vi "SerialPort.Get Status.vi"(8 "error in (no error)":errorcluster, 11 "SerialPort in":refnum<class "SerialPort.lvclass">) -> (0 "error out":errorcluster, 2 "State":T1, 3 "SerialPort out":refnum<class "SerialPort.lvclass">)   [LabVIEW 2018, in "SerialPort.lvclass"]
uses:
  SerialPort.lvclass
  Controls/SerialPort.Status Enum.ctl
  SerialPort.lvclass/SerialPort.ctl
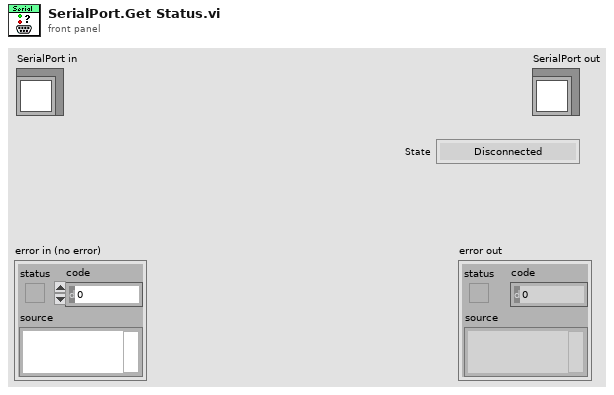
[diagram p1: front panel]
types:
  T1 = typedef "SerialPort.Status Enum.ctl" = enum16{"Disconnected", "Connecting", "Connected"}
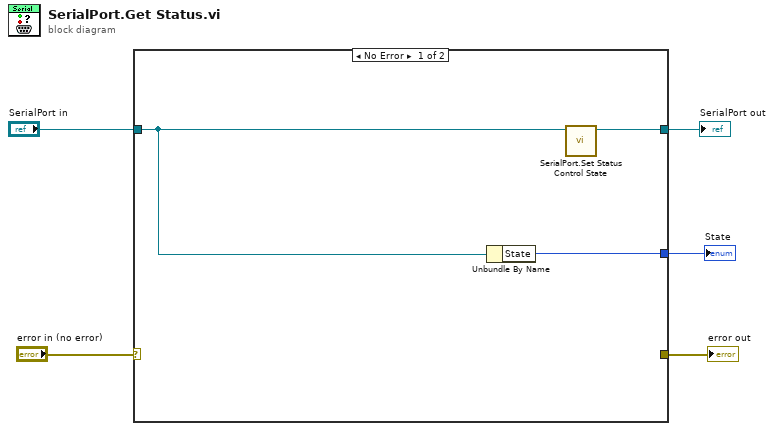
[diagram p0: block diagram]
diagram:
  n1 = case shown="No Error" "error in (no error)" {
    selector: "error in (no error)" -> [_ w10]
    tunnel: [_ w10] -> w4
    tunnel: [w8 w9] -> w2
    tunnel: "SerialPort in" -> [w6 w9]
    tunnel: [w7 _] -> w1
    frame No Error {
      n2 = Unbundle By Name(w6) -> ("State"=w7:T1)
      n3 = call "SerialPort.Set Status Control State.vi"("SerialPort in"=w6) -> ("SerialPort out"=w8:refnum<class "SerialPort.lvclass">)  [unwired: 9 in, 1 out]
    }
    frame Error {
    }
  }
  "error out" <- w4
  "SerialPort out" <- w2
  "State" <- w1
